vi "Destroy.vi"(8 "Error In":errorcluster, 11 "reference in":refnum<class "BoldDecorator.lvclass">) -> (0 "Error Out":errorcluster, 3 "reference out":refnum<class "BoldDecorator.lvclass">)   [LabVIEW 2024, in "BoldDecorator.lvclass"]
uses:
  BoldDecorator.lvclass
  TextDecorator/TextDecorator.lvclass
  AbstractText/AbstractText.lvclass
  BoldDecorator.lvclass/BoldDecorator.ctl
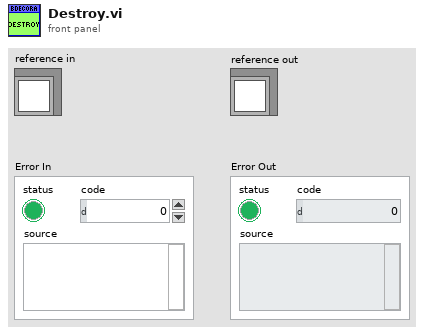
[diagram p1: front panel]
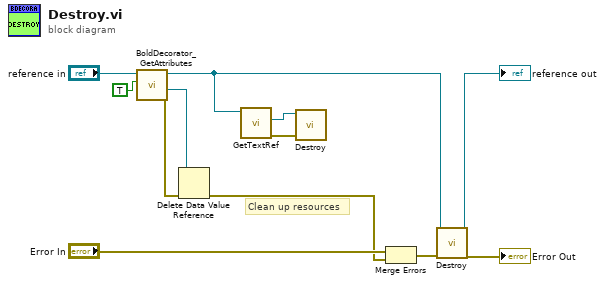
[diagram p0: block diagram]
diagram:
  # "Clean up resources"
  n1 = call "BoldDecorator_GetAttributes.vi"("OnlyGetDvrReference(False)"=TRUE, "reference in"="reference in") -> ("Error Out"=w10:errorcluster, "DataRef"=w9:refnum<data-value>, "reference out"=w3:refnum<class "BoldDecorator.lvclass">)  [unwired: 6 in, 1 out]
  n2 = Delete Data Value Reference(data value reference=w9, error in=w10) -> (error out=w7:errorcluster)  [unwired: 1 out]
  n3 = call-dynamic "GetTextRef.vi"("reference in"=w3) -> ("Error Out"=w2:errorcluster, "TextRef"=w1:refnum<class "AbstractText.lvclass">)  [unwired: 8 in, 1 out]
  n4 = call-dynamic "Destroy.vi"("Error In"=w2, "reference in"=w1) -> ()  [unwired: 8 in, 2 out]
  n5 = Merge Errors("Error In", w7) -> (w12:errorcluster)
  n6 = call-parent "Destroy.vi"("Error In"=w12, "reference in"=w3) -> ("Error Out"=→"Error Out":errorcluster, "reference out"=→"reference out":refnum<class "BoldDecorator.lvclass">)  [unwired: 8 in]
